vi "BlendSuggestionsToGoStraight.vi"(9 "BalanceRudderSailSuggestion":T1 {"MainSailSuggestion" min=0.0 max=1.0; "JibSailSuggestion" min=0.0 max=1.0}, 10 "LuffToSailSuggestion":T1 {"MainSailSuggestion" min=0.0 max=1.0; "JibSailSuggestion" min=0.0 max=1.0}, 11 "WindToSailLookup":T1 {"MainSailSuggestion" min=0.0 max=1.0; "JibSailSuggestion" min=0.0 max=1.0}) -> (3 "BlendedGoStraightSailSetting":T1 {"MainSailSuggestion" min=0.0 max=1.0; "JibSailSuggestion" min=0.0 max=1.0})   [LabVIEW 2012]
doc: "This VI takes in suggestions for\n1) Simple sail lookup by Point of Sail\n2) How to move the sails to balance the rudder\n3) How to move the sails to stop luffing\n\nThis VI is intended to generally pass through #1 unimpeded, but gradually filter in the advice from #2 and #3 over time. The mechanism for this will be either increasing the gain of suggestions (2, 3) as the boat nears 'cruising' velocity or indcreasing the gain as a function of the time spent in the 'go straight' boat state."
uses:
  Data/TypeDefs/Sail Set Suggestions.ctl
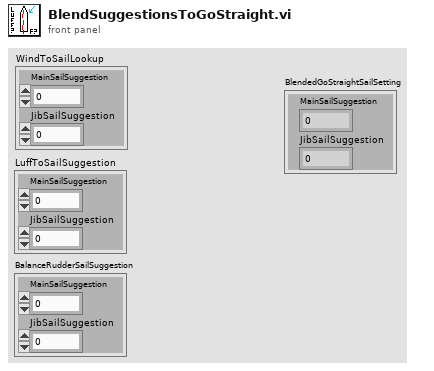
[diagram p1: front panel]
types:
  T1 = typedef "Sail Set Suggestions.ctl" = cluster{"MainSailSuggestion":dbl, "JibSailSuggestion":dbl}
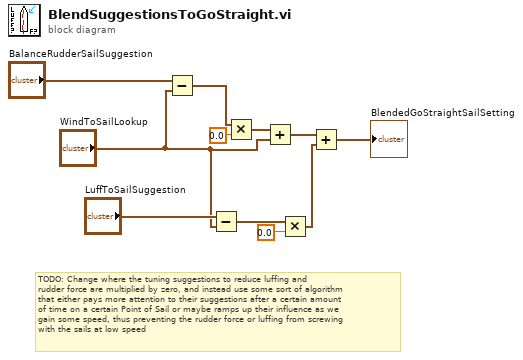
[diagram p0: block diagram]
diagram:
  # "TODO: Change where the tuning suggestions to reduce luffing and\nrudder force are multiplied by zero, and instead use some sort of algorithm\nthat either pays more attention to their suggestions after a certain amount\nof time on a certain Point of Sail or maybe ramps up their influence as we\ngain some speed, thus preventing the rudder force or luffing from screwing\nwith the sails at low speed"
  n1 = Subtract(x="BalanceRudderSailSuggestion", y="WindToSailLookup") -> (x-y=w10:T1)
  n2 = Subtract(x="LuffToSailSuggestion", y="WindToSailLookup") -> (x-y=w9:T1)
  n3 = Multiply(x=w10, y=0.0) -> (x*y=w2:T1)
  n4 = Add(x=w2, y="WindToSailLookup") -> (x+y=w11:T1)
  n5 = Multiply(x=w9, y=0.0) -> (x*y=w6:T1)
  n6 = Add(x=w11, y=w6) -> (x+y=→"BlendedGoStraightSailSetting":T1)
